vi "niFpgaPeriodTemplateNoInterpolate.vi"(0 "input data":fxp<+/-,16,16>, 1 "reset":bool, 5 "threshold level":fxp<+/-,16,16>, 7 "hysteresis":fxp<+/-,16,16>, 9 "direction":u8(ring) items=["falling", "rising"]) -> (4 "period (samples)":fxp<+,32,16>, 6 "timeout":bool, 8 "crossing":bool, 10 "output valid":bool)   [LabVIEW 2017]
uses:
  <vilib>/Platform/TimedLoop/XDataNode/timing_clust.ctl
  <vilib>/Platform/TimedLoop/XDataNode/nitl_modes.ctl
  <vilib>/Platform/TimedLoop/XDataNode/wakeup.ctl
  <vilib>/Platform/TimedLoop/XDataNode/XDataNode.xnode
  <vilib>/Platform/TimedLoop/XDataNode/XDNodeRunTimeDep.lvlib
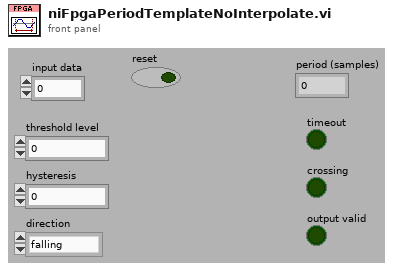
[diagram p1: front panel]
types:
  T1 = typedef "XDNodeRunTimeDep.lvlib/timing_clust.ctl" = cluster{"Expected End [f-1]":u64, "Actual End [f-1]":u64, "Finished Late? [f-1]":bool, "Expected End [i-1]":u64, "Actual End [i-1]":u64, "Finished Late? [i-1]":bool, "Expected Start [i]":u64, "Actual Start [i]":u64, "Expected Start [f]":u64, "Actual Start [f]":u64, "Source Name":string, "Structure Name":string, "Period":i64, "Deadline":i64, "Offset":i64, "Start":i64, "Priority":i32, "Timeout":i32, "Mode":T2, "Wakeup Reason":T3, "Error":errorcluster, "Source Type":string, "Secondary Source Type":string, "Global End Time":u64, "Global Start Time":u64, "Frame Duration":u64, "Iteration Duration":u64, "Assigned CPU":i32, "I/O Scan Engine Mode":u32}
  T2 = typedef "XDNodeRunTimeDep.lvlib/nitl_modes.ctl" = enum32{"No Change", "Process missed periods, maintain original phase", "Discard missed periods, maintain original phase", "Process missed periods, ignore original phase", "Discard missed periods, ignore original phase"}
  T3 = typedef "XDNodeRunTimeDep.lvlib/wakeup.ctl" = enum32{"Normal", "Aborted", "Asynchronous wakeup", "Timing source error", "Timed loop error", "Timeout"}
  T4 = typedef "niFPGA Threshold Crossing State.ctl" = cluster{"level":bool[], "rising?":bool, "hi hyst met?":bool, "lo hyst met?":bool, "gt threshold":bool, "lt threshold":bool}
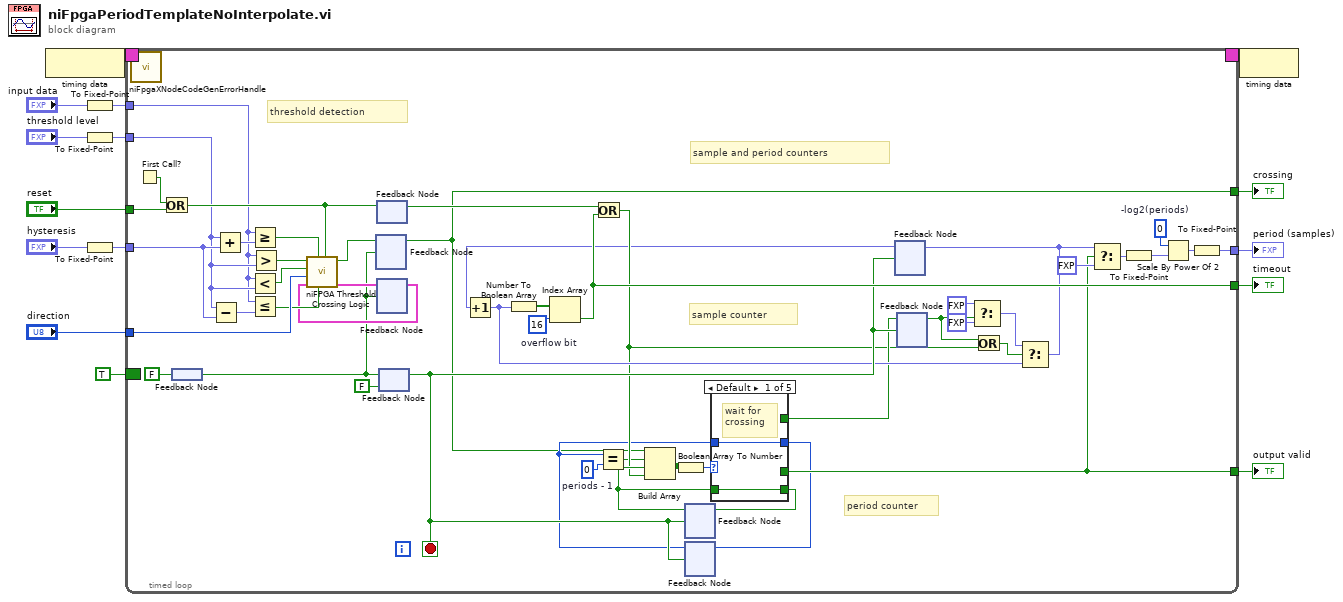
[diagram p0: block diagram]
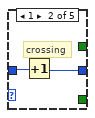
[diagram p2: hidden frame]
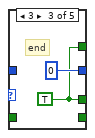
[diagram p3: hidden frame]
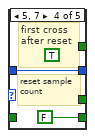
[diagram p4: hidden frame]
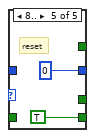
[diagram p5: hidden frame]
diagram:
  n1 = node-c288() -> (w14:T1)
  n2 = To Fixed-Point(number="input data") -> (fixed-point=w3:fxp<+/-,16,16>)  [unwired: 1 in]
  n3 = To Fixed-Point(number="threshold level") -> (fixed-point=w2:fxp<+/-,16,16>)  [unwired: 1 in]
  n4 = To Fixed-Point(number="hysteresis") -> (fixed-point=w1:fxp<+/-,16,16>)  [unwired: 1 in]
  n5 = timed-loop "SCTL" {
    tunnel: [w38] -> w5
    tunnel: [w39] -> w15
    timing: w14 -> [_]
    timing-out: [_] -> w13
    tunnel: [w65] -> w12
    tunnel: w3 -> [w48]
    tunnel: "direction" -> [w57]
    tunnel: w2 -> [w50]
    tunnel: w1 -> [w64]
    tunnel: "reset" -> [w63]
    border: TRUE -> [_]
    tunnel: [w17] -> w4
    stop <- w49 stop-if-true
    w21 = u16 0  # periods - 1
    w30 = 16  # overflow bit
    w44 = i16 0  # -log2(periods)
    # "period counter"
    # "sample counter"
    # "sample and period counters"
    # "threshold detection"
    n6 = First Call?() -> (First Call?: T/F=w47:bool)
    n7 = Or(x=w47, y=w63) -> (x .or. y?=w55:bool)
    n8 = feedback-in #1(FALSE) -> ()
    n9 = feedback #1() -> (w18:bool)
    n10 = Subtract(x=w50, y=w64) -> (x-y=w62:fxp<+/-,17,17>)
    n11 = Add(x=w50, y=w64) -> (x+y=w61:fxp<+/-,17,17>)
    n12 = Greater Or Equal?(x=w48, y=w61) -> (x >= y?=w60:bool)
    n13 = Less?(x=w48, y=w50) -> (x < y?=w58:bool)
    n14 = Less Or Equal?(x=w48, y=w62) -> (x <= y?=w56:bool)
    n15 = Greater?(x=w48, y=w50) -> (0:w59:bool)
    n16 = feedback #2() -> (w17:bool)  [unwired: 1 in]
    n17 = feedback-in #3(w55) -> ()
    n18 = feedback #3() -> (w46:bool)  [unwired: 1 in]
    n19 = feedback #4() -> (w53:T4)  [unwired: 1 in]
    n20 = call <vilib>:"niFPGA Threshold Crossing Logic.vi"("reset"=w55, "le low ref"=w56, "ge high ref"=w60, "state in"=w53, "direction"=w57, "lt threshold"=w58, "gt threshold"=w59) -> ("state out"=w54:T4, "crossing"=w52:bool)  [unwired: 3 in]
    n21 = feedback-in #2(w52, w18) -> ()
    n22 = feedback-in #4(w54, w18) -> ()
    n23 = feedback-in #5(w18) -> ()
    n24 = feedback #5(FALSE) -> (w49:bool)
    n25 = feedback #6() -> (w33:bool)  [unwired: 1 in]
    n26 = feedback #7() -> (w22:u16)  [unwired: 1 in]
    n27 = Equal?(x=w22, y=w21) -> (x = y?=w23:bool)
    n28 = feedback #8() -> (w19:fxp<+,25,25>)  [unwired: 1 in]
    n29 = Increment(x=w19) -> (x+1=w32:fxp<+,25,25>)
    n30 = Number To Boolean Array(number=w32) -> (Boolean array=w31:bool[])
    n31 = Index Array(array=w31, index=w30) -> (element=w65:bool)
    n32 = Or(x=w46, y=w65) -> (x .or. y?=w25:bool)
    n33 = Build Array(w17, w23, w33, w25) -> (w37:bool[])
    n34 = Boolean Array To Number(Boolean array=w37) -> (number=w36:u8)
    n35 = case shown="Default" w36 {
      tunnel: [w66 _ _ FALSE TRUE] -> w35
      tunnel: w22 -> [w67 w69 _ w74 _]
      tunnel: [w67 w68 u16 0 w74 u16 0] -> w34
      tunnel: w33 -> [w66 _ _ _ _]
      tunnel: [_ _ w70 _ _] -> w39
      tunnel: [_ _ w70 TRUE _] -> w26
      frame Default {
        # "wait for crossing"
      }
      frame 1 {
        # "crossing"
        n36 = Increment(x=w69) -> (x+1=w68:u16)
      }
      frame 3 {
        w70 = TRUE
        # "end"
      }
      frame 5, 7 {
        # "reset sample count"
        # "first cross after reset"
      }
      frame 8.. {
        # "reset"
      }
    }
    n37 = feedback-in #6(w35, w49) -> ()
    n38 = feedback-in #7(w34, w49) -> ()
    n39 = feedback #9() -> (w20:bool)  [unwired: 1 in]
    n40 = feedback-in #9(w26, w49) -> ()
    n41 = Select(t=fxp<+,25,25> 1.0, s=w20, f=fxp<+,25,25> 0.0 ("t")) -> (s? t:f=w27:fxp<+,25,25>)
    n42 = Or(x=w20, y=w25) -> (x .or. y?=w24:bool)
    n43 = Select(t=w27, s=w24, f=w32) -> (s? t:f=w40:fxp<+,25,25>)
    n44 = feedback-in #8(w40, w49) -> ()
    n45 = Select(t=w40, s=w39, f=fxp<+,25,25> 0.0) -> (s? t:f=w45:fxp<+,25,25>)
    n46 = To Fixed-Point(number=w45) -> (fixed-point=w41:fxp<+/-,42,26>)  [unwired: 1 in]
    n47 = Scale By Power Of 2(n=w44, x=w41) -> (x*2^n=w42:fxp<+/-,42,26>)
    n48 = To Fixed-Point(number=w42) -> (fixed-point=w38:fxp<+,32,16>)  [unwired: 1 in]
  }
  "output valid" <- w15
  "period (samples)" <- w5
  "timeout" <- w12
  "crossing" <- w4
  n49 = call <vilib>:"niFpgaXNodeCodeGenErrorHandle.vi"() -> ()  [unwired: 1 in]
  n50 = node-c288(w13) -> ()
